vi "Get Veristand Versions.vi"(8 "error in (no error)":errorcluster) -> (0 "error out":errorcluster, 3 "Versions":cluster{"String":string, "Value":string}[](array[cluster]))   [LabVIEW 2019, in "Configuration Tool.lvlib"]
uses:
  Configuration Tool.lvlib
  <vilib>/Utility/sysdir.llb/System Directory Type.ctl
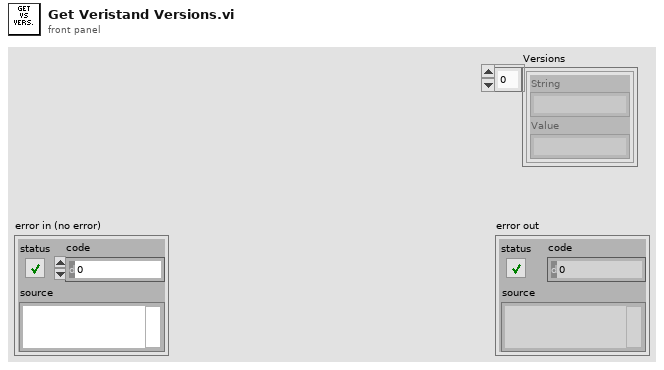
[diagram p1: front panel]
types:
  T1 = typedef "System Directory Type.ctl" = i32
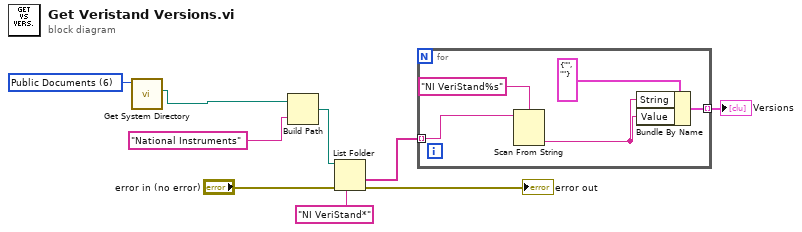
[diagram p0: block diagram]
diagram:
  w5 = T1 6 items=["User Home"=0, "User Desktop"=1, "User Documents"=2, "User Application Data"=3, "User Preferences"=4, "User Temporary"=5, "Public Documents"=6, "Public Application Data"=7, "Public Preferences"=8, "Public Cache"=13, "System Core Libraries"=9, "System Installed Libraries"=10, "Application Files"=11, "Boot Volume Root"=12] ("system directory type")
  n1 = call <vilib>:"Get System Directory.vi"("system directory type"=w5) -> ("system directory"=w4:path)  [unwired: 10 in]
  n2 = Build Path(base path=w4, name or relative path="National Instruments") -> (appended path=w2:path)
  n3 = List Folder(path=w2, pattern="NI VeriStand*", error in="error in (no error)") -> (folder names=w7:string[], error out=→"error out":errorcluster)  [unwired: 1 in, 2 out]
  n4 = for {
    tunnel: w7 -> [w14] mode=indexing
    tunnel: [w10] -> w1 mode=indexing
    n5 = Scan From String(format string="NI VeriStand%s", input string=w14) -> (output 1=w11:string)  [unwired: 3 in, 3 out]
    n6 = Bundle By Name(cluster=cluster{"String":string, "Value":string} {"String"="", "Value"=""} ("Cluster"), "String"=w11, "Value"=w11) -> (w10:cluster{"String":string, "Value":string})
  }
  "Versions" <- w1
